vi "check arrays.vi"(10 "array 2":cdb[](array[numeric]), 11 "array 1":cdb[](array[numeric])) -> (0 "error out":errorcluster)   [LabVIEW 2020]
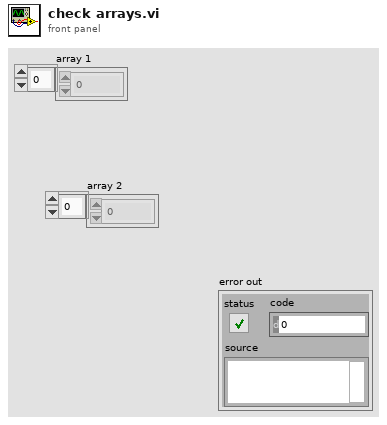
[diagram p1: front panel]
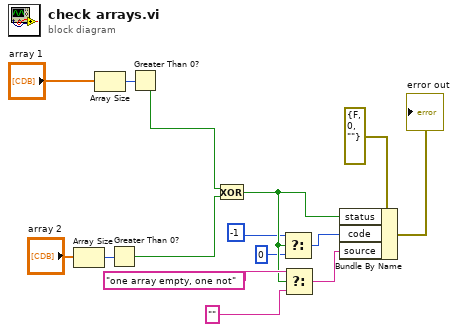
[diagram p0: block diagram]
diagram:
  n1 = Array Size(array="array 2") -> (size(s)=w3:i32)
  n2 = Array Size(array="array 1") -> (size(s)=w2:i32)
  n3 = Greater Than 0?(x=w3) -> (x > 0?=w5:bool)
  n4 = Greater Than 0?(x=w2) -> (x > 0?=w4:bool)
  n5 = Exclusive Or(1:w5, 2:w4) -> (0:w11:bool)
  n6 = Select(t=-1 ("code"), s=w11, f=0) -> (s? t:f=w7:i32)
  n7 = Select(t="one array empty, one not", s=w11, f="" ("source")) -> (s? t:f=w10:string)
  n8 = Bundle By Name(cluster=errorcluster {"status"=FALSE, "code"=0, "source"=""} ("error out"), "status"=w11, "code"=w7, "source"=w10) -> (→"error out":errorcluster)
